vi "RayTriDirCheck.vi"(8 "Normal":dbl[](array[numeric]), 9 "TriVertex":dbl[](array[numeric]), 10 "Dir":dbl[](array[numeric]), 11 "P0":dbl[](array[numeric])) -> (1 "w":dbl[](array[numeric]), 2 "r":dbl, 3 "I":dbl[](array[numeric]))   [LabVIEW 2014]
uses:
  <vilib>/Analysis/baseanly.llb/Real Dot Product.vi
  <vilib>/Analysis/NI_AALBase.lvlib
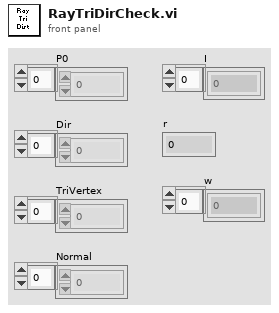
[diagram p1: front panel]
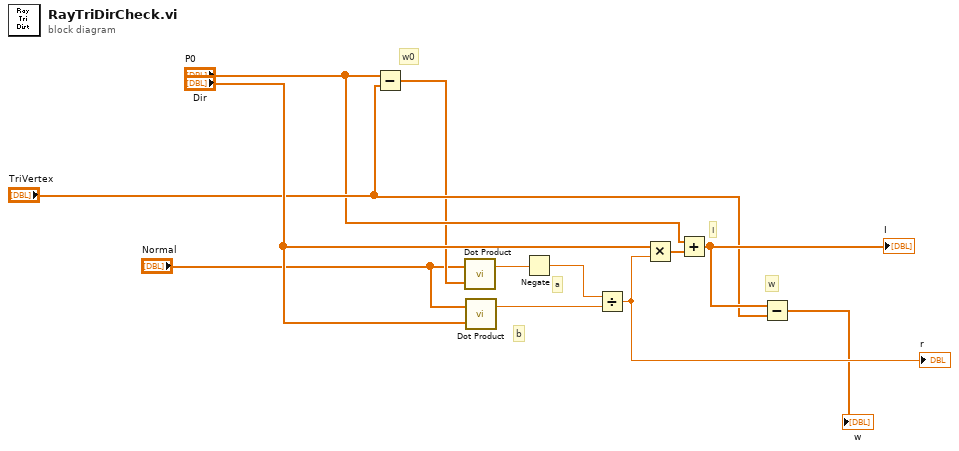
[diagram p0: block diagram]
diagram:
  # "I"
  # "w"
  # "b"
  # "a"
  # "w0"
  n1 = Subtract(x="P0", y="TriVertex") -> (x-y=w5:dbl[])
  n2 = call-poly <vilib>:"Dot Product.vi"("Y Vector"=w5, "X Vector"="Normal") -> ("X * Y"=w1:dbl)  [unwired: 1 out]
  n3 = call-poly <vilib>:"Dot Product.vi"("Y Vector"="Dir", "X Vector"="Normal") -> ("X * Y"=w4:dbl)  [unwired: 1 out]
  n4 = Negate(x=w1) -> (-x=w3:dbl)
  n5 = Divide(x=w3, y=w4) -> (x/y=w12:dbl)
  "r" <- w12
  n6 = Multiply(x="Dir", y=w12) -> (x*y=w6:dbl[])
  n7 = Add(x="P0", y=w6) -> (x+y=w10:dbl[])
  "I" <- w10
  n8 = Subtract(x=w10, y="TriVertex") -> (x-y=→"w":dbl[])
